vi "asset.property_count.vi"(8 "error in":errorcluster, 11 "object_in":refnum<class "Asset.lvclass">) -> (0 "error out":errorcluster, 3 "object_out":refnum<class "Asset.lvclass">)   [LabVIEW 2020, in "Asset.lvclass"]
doc: "Returns the number of properties on the asset."
uses:
  Asset.lvclass
  Asset.lvclass/Asset.ctl
  client.lvlib
panel:
  out "function return":i32
  out "out_count out":u32
  in  "out_count":u32
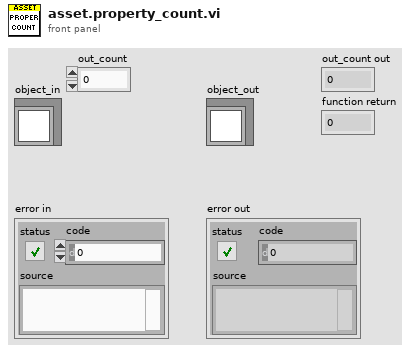
[diagram p1: front panel]
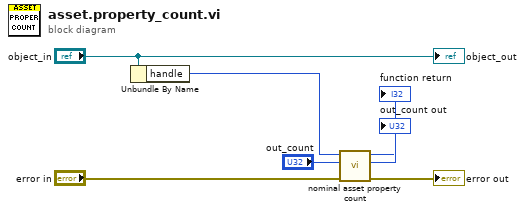
[diagram p0: block diagram]
diagram:
  n1 = Unbundle By Name("object_in") -> ("handle"=w5:i32)
  n2 = call "nominal asset property count.vi"("error in (no error)"="error in", "out_count"="out_count", "asset"=w5) -> ("error out"=→"error out":errorcluster, "out_count out"=→"out_count out":u32, "function return"=→"function return":i32)  [unwired: 6 in]
  "object_out" <- "object_in"
